vi "tempconfig.vi"(1 "Temp Config in":T1, 2 "command":string) -> (0 "Temp Config out":T1)   [LabVIEW 2010]
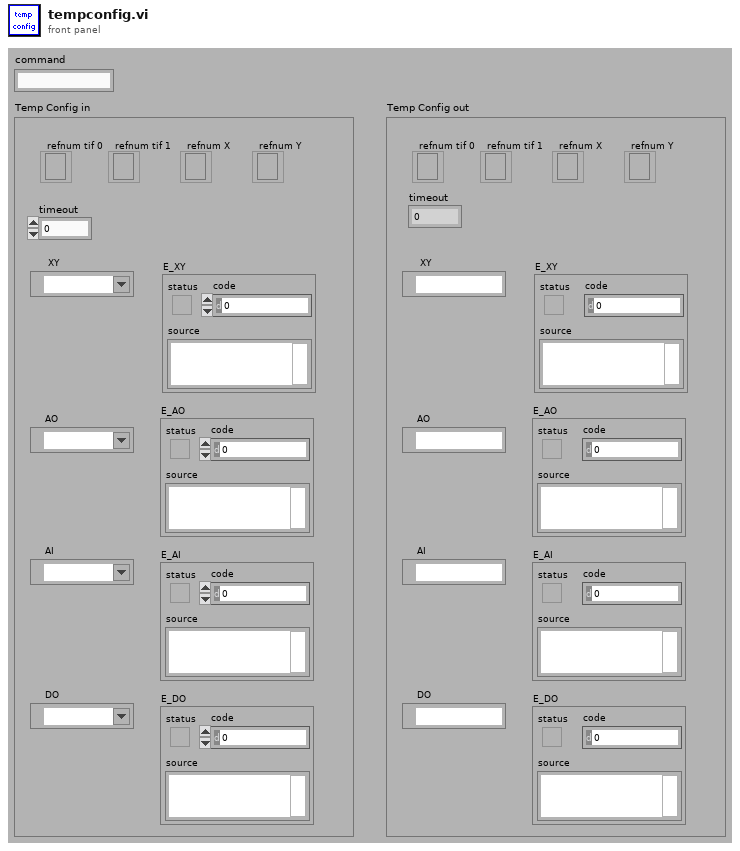
[diagram p1: front panel]
types:
  T1 = cluster{"refnum tif 0":refnum<file>, "refnum tif 1":refnum<file>, "refnum X":refnum<file>, "refnum Y":refnum<file>, "timeout":dbl, " XY":refnum<k21>, "AO":refnum<k21>, "AI":refnum<k21>, "DO":refnum<k21>, "E_XY":errorcluster, "E_AO":errorcluster, "E_AI":errorcluster, "E_DO":errorcluster}
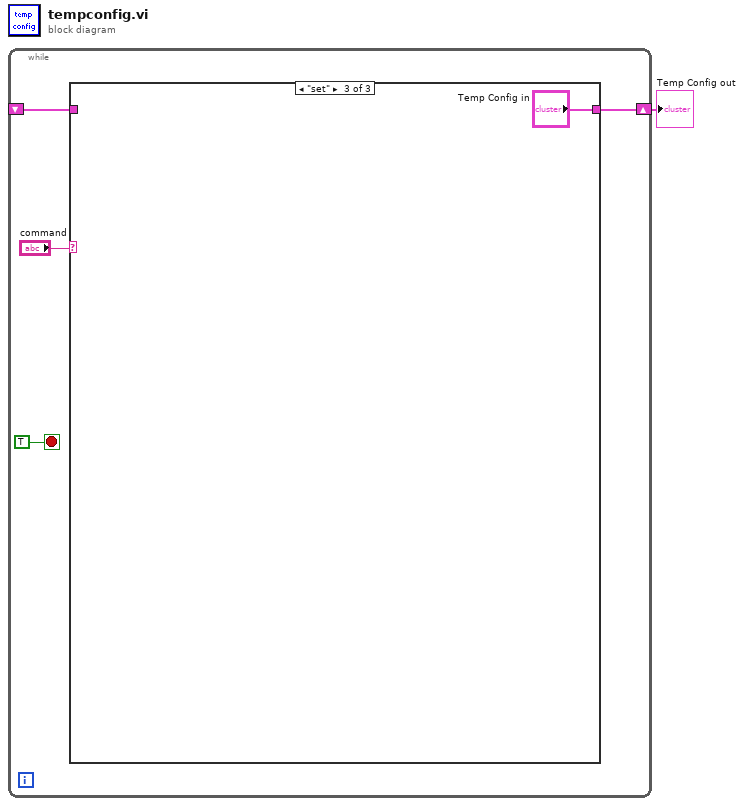
[diagram p0: block diagram]
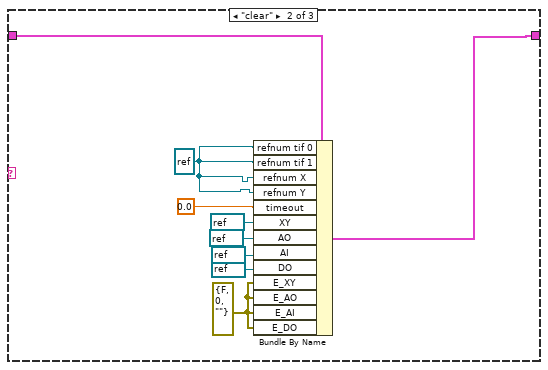
[diagram p3: hidden frame]
diagram:
  n1 = while {
    shift-right: [w3] -> w1
    shift-left: _ -> [w2]
    stop <- TRUE stop-if-true
    n2 = case shown="\"set\"" "command" {
      tunnel: [w6 w8 "Temp Config in"] -> w3
      tunnel: w2 -> [w6 w15 _]
      frame "get", Default {
      }
      frame "clear" {
        w7 = errorcluster {"status"=FALSE, "code"=0, "source"=""} ("E_AI")
        w14 = refnum<file> refnum ("refnum tif 1")
        n3 = Bundle By Name(cluster=w15, "refnum tif 0"=w14, "refnum tif 1"=w14, "refnum X"=w14, "refnum Y"=w14, "timeout"=0.0, "XY"=refnum<k21> refnum, "AO"=refnum<k21> refnum ("XY"), "AI"=refnum<k21> refnum ("XY"), "DO"=refnum<k21> refnum ("XY"), "E_XY"=w7, "E_AO"=w7, "E_AI"=w7, "E_DO"=w7) -> (w8:T1)
      }
      frame "set" {
      }
    }
  }
  "Temp Config out" <- w1
